vi "ROI_Process Snippet with ROI Information.vi"(8 "error in (no error)":errorcluster, 11 "ROI Snippet":T1) -> (0 "error out":errorcluster, 2 "ROI Information":dbl)   [LabVIEW 2012]
uses:
  <vilib>/vision/Image Controls.llb/IMAQ Image.ctl
  <vilib>/vision/NI_Vision_Development_Module.lvlib
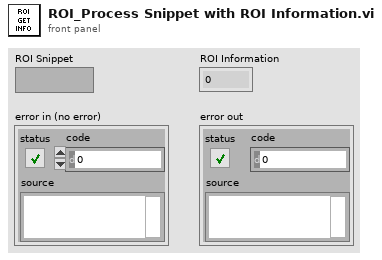
[diagram p1: front panel]
types:
  T1 = typedef "IMAQ Image.ctl" = refnum<image>
  T2 = cluster{"Mean Value":sgl, "Standard Variation":sgl, "Minimal Value":sgl, "Maximal Value":sgl, "Area (calibrated)":sgl, "Area (pixels)":u32, "%":sgl, "Calibration Valid":bool}
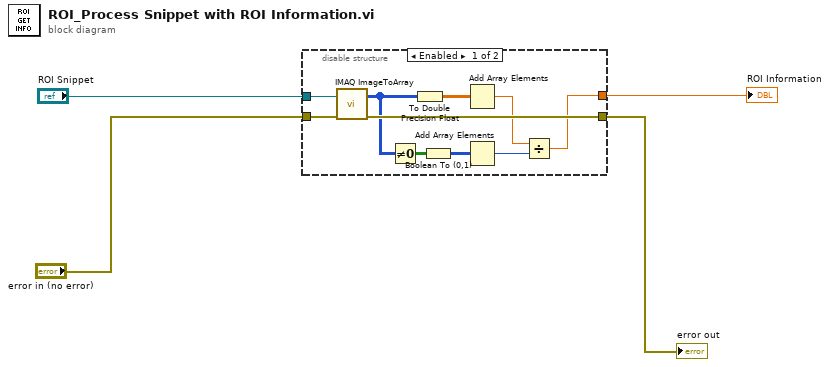
[diagram p0: block diagram]
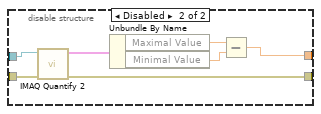
[diagram p2: hidden frame]
diagram:
  n1 = disable-structure shown="Enabled" {
    disable-tunnel: "ROI Snippet" -> [w14 w21]
    disable-tunnel: [w5 w15] -> w1
    disable-tunnel: "error in (no error)" -> [w12 w20]
    disable-tunnel: [w11 w19] -> w4
    frame Enabled {
      n2 = call "IMAQ ImageToArray"("error in (no error)"=w12, "Image"=w14) -> ("error out"=w11:errorcluster, "Image Pixels (I16)"=w10:i16[][])  [unwired: 2 in, 3 out]
      n3 = Not Equal To 0?(x=w10) -> (x != 0?=w9:bool[][])
      n4 = To Double Precision Float(number=w10) -> (double precision float=w13:dbl[][])
      n5 = Boolean To (0,1)(Boolean=w9) -> (0, 1=w8:i16[][])
      n6 = Add Array Elements(numeric array=w13) -> (sum=w6:dbl)
      n7 = Add Array Elements(numeric array=w8) -> (sum=w7:i16)
      n8 = Divide(x=w6, y=w7) -> (x/y=w5:dbl)
    }
    frame Disabled {
      n9 = call "IMAQ Quantify 2"("error in (no error)"=w20, "Image"=w21) -> ("error out"=w19:errorcluster, "Global Report"=w18:T2)  [unwired: 7 in, 1 out]
      n10 = Unbundle By Name(w18) -> ("Maximal Value"=w17:sgl, "Minimal Value"=w16:sgl)
      n11 = Subtract(x=w17, y=w16) -> (x-y=w15:sgl)
    }
  }
  "error out" <- w4
  "ROI Information" <- w1
